vi "(alter)Mecanum Steering.vi"() -> ()   [LabVIEW 2015]
doc: "This example shows how to use the Steering VIs to define and simulate a dynamic model of a three-wheeled omnidirectional robot on a smooth surface."
uses:
  Program Files (x86)/National Instruments/LabVIEW 2015/examples/robotics/Steering/3D Omni Robot/Robot Position.ctl
  <vilib>/robotics/Steering/Wheel/Wheel Parameters.ctl
  <vilib>/robotics/Steering/Wheel/Rotation Direction.ctl
  <vilib>/Simulation/Scripting/Companion Diagram/SimConfigNode/SimParams.ctl
  <vilib>/Simulation/Scripting/Companion Diagram/SimConfigNode/_simSolvers.ctl
  <vilib>/Simulation/Implementation/Shared/SIMSCR Execution Mode.ctl
  <vilib>/Platform/TimedLoop/XDataNode/timing_clust.ctl
  <vilib>/Platform/TimedLoop/XDataNode/nitl_modes.ctl
  <vilib>/Platform/TimedLoop/XDataNode/wakeup.ctl
  <vilib>/Simulation/Param Hierarchy/Typedefs/SIMPH Param Control Actions.ctl
  <vilib>/Simulation/Implementation/Shared/NILVSim_ParamChanged.vi
  <vilib>/Simulation/Implementation/Shared/NILVSim_FinishedLate.vi
  <vilib>/Simulation/Implementation/Shared/NILVSIM_BeginStep.vi
  <vilib>/Simulation/Utility/Implementation/SIM Halt.vi
  <vilib>/Simulation/Implementation/Shared/NILVSim_Manager.vi
  <vilib>/Utility/error.llb/Clear Errors.vi
  <vilib>/Simulation/Implementation/Shared/NILVSim_FinalizeModel.vi
  <vilib>/Analysis/coordinate.llb/2D Cartesian Coordinate Rotation.vi
  <vilib>/Analysis/coordinate.llb/2D Cartesian Coordinate Rotation (Scalar).vi
  <vilib>/robotics/Steering/Omnidirectional Wheel/Create Omnidirectional Wheel.vi
  <vilib>/robotics/Steering/Steering Frame/Create User Defined Steering Frame.vi
  <vilib>/Simulation/Implementation/Shared/SIM Unbundle Sim Info.vi
  <vilib>/Simulation/Implementation/Shared/SIMSH Read Queue.vi
  <vilib>/Simulation/Implementation/Shared/NILVSim_Initialize.vi
  <vilib>/Simulation/Utility/Implementation/NILVSim Get Time and IsAcceptedStep.vi
  <vilib>/Simulation/Implementation/Shared/NILVSim_GetModelError.vi
  <vilib>/Simulation/Implementation/Shared/SIM Bundle Sim Info.vi
  <vilib>/robotics/Steering/Steering Frame/Apply Steering Frame Velocity to Motors.vi
  <vilib>/robotics/Steering/Steering Frame/Get Steering Frame Velocity from Motors.vi
  <vilib>/Simulation/Scripting/Companion Diagram/SimConfigNode/SimDog.xnode
  Program Files (x86)/National Instruments/LabVIEW 2015/examples/robotics/Steering/3D Omni Robot/Omni Robot Model.vi
  <vilib>/Platform/TimedLoop/XDataNode/XDataNode.xnode
  <vilib>/Simulation/Implementation/XNodeFramework/SimXNode/SimX.xnode
  <vilib>/robotics/Steering/Steering Frame/NI_Robotics_Steering Frame.lvclass
  <vilib>/robotics/Steering/Wheel/NI_Robotics_Wheel.lvclass
  <vilib>/robotics/Steering/Omnidirectional Wheel/NI_Robotics_Omnidirectional Wheel.lvclass
  <vilib>/Platform/TimedLoop/XDataNode/XDNodeRunTimeDep.lvlib
  <vilib>/Simulation/Implementation/Shared/NI_SIM_Implementation.lvlib
panel:
  in  "目標in 2":T1={"起始"=0.0, "終點"=200.0, "max speed(估算)"=80.0, "dt"=10.0}
  out "距離曲線(cm) 2":dbl[](array[numeric])
  out "次數 2":i32
  out "speed曲線(cm/s) 2":dbl[](array[numeric])
  out "speed曲線(cm/s)":dbl[](array[numeric])
  out "次數":i32
  out "距離曲線(cm)":dbl[](array[numeric])
  in  "目標in":T1={"起始"=0.0, "終點"=200.0, "max speed(估算)"=80.0, "dt"=10.0}
  out "Waveform Chart 2":T2(graph)
  out "xy theta":T2(graph)
  in  "Velocity":T3(ring)
  in  "reset":bool
  in  "stop":bool
  in  "Angular Velocity (rad/s)":dbl(slide) min=-7.0 max=7.0 scale=-7.0..7.0
  out "Angular Velocity Feedback":dbl(slide) scale=1.0..-1.0
  in  "Y Velocity (cm/s)":dbl(slide) min=-100.0 max=100.0 scale=-100.0..100.0
  out "Y Velocity Feedback":dbl(slide) scale=-1.0..1.0
  in  "X Velocity (cm/s)":dbl(slide) min=-100.0 max=100.0 scale=-100.0..100.0
  out "X Velocity Feedback":dbl(slide) scale=-1.0..1.0
  out "motor states":dbl[](array[numeric]) format="%#.3f"
  in  "motor setpoints":dbl[](array[numeric])=[0.0, 0.0, 0.0] format="%#.3f"
  out "complete":bool
  out "robot position":T4 {"ccw wheel angles" format="%#.3f"; "global theta" format="%#.3f"; "global y" format="%#.3f"; "global x" format="%#.3f"}
  out "3D Picture":refnum<vi>(3d-picture)
  # "This VI simulates the steering of a three-wheeled omnidirectional robot on a smooth surface.\n\n1. Run the VI, then move the sliders to control the forward, lateral, and angular velocity components of the robot.\n\n2. Press the Reset Position button to move the robot back to its starting position."
types:
  T1 = cluster{"起始":dbl, "終點":dbl, "max speed(估算)":dbl, "dt":dbl}
  T2 = cluster{"motor states[0]":dbl, "motor states[1]":dbl, "motor states[2]":dbl, "motor states[3]":dbl, "motor states[4]":dbl, "motor states[5]":dbl, "motor states[6]":dbl, "motor states[7]":dbl, "motor states[8]":dbl}
  T3 = enum16{"Relative to Steering Frame", "Relative to Global Frame"}
  T4 = typedef "Robot Position.ctl" = cluster{"global x":dbl, "global y":dbl, "global theta":dbl, "ccw wheel angles":dbl[]}
  T5 = typedef "NI_Robotics_Wheel.lvclass/Rotation Direction.ctl" = u16
  T6 = typedef "NI_Robotics_Wheel.lvclass/Wheel Parameters.ctl" = cluster{"wheel radius":dbl, "gear ratio":dbl, "forward rotation direction":T5}
  T7 = cluster{"[0]":dbl, "[1]":dbl, "[2]":dbl, "[3]":dbl, "[4]":dbl, "[5]":dbl, "[6]":dbl, "[7]":dbl, "[8]":dbl}
  T8 = typedef "SIMSCR Execution Mode.ctl" = enum16{"Simulate to Completion", "Single Time-Step Simulation (Fixed Step Only)"}
  T9 = typedef "XDNodeRunTimeDep.lvlib/timing_clust.ctl" = cluster{"Expected End [f-1]":u64, "Actual End [f-1]":u64, "Finished Late? [f-1]":bool, "Expected End [i-1]":u64, "Actual End [i-1]":u64, "Finished Late? [i-1]":bool, "Expected Start [i]":u64, "Actual Start [i]":u64, "Expected Start [f]":u64, "Actual Start [f]":u64, "Source Name":string, "Structure Name":string, "Period":i64, "Deadline":i64, "Offset":i64, "Start":i64, "Priority":i32, "Timeout":i32, "Mode":T10, "Wakeup Reason":T11, "Error":errorcluster, "Source Type":string, "Secondary Source Type":string, "Global End Time":u64, "Global Start Time":u64, "Frame Duration":u64, "Iteration Duration":u64, "Assigned CPU":i32, "I/O Scan Engine Mode":u32}
  T10 = typedef "XDNodeRunTimeDep.lvlib/nitl_modes.ctl" = enum32{"No Change", "Process missed periods, maintain original phase", "Discard missed periods, maintain original phase", "Process missed periods, ignore original phase", "Discard missed periods, ignore original phase"}
  T11 = typedef "XDNodeRunTimeDep.lvlib/wakeup.ctl" = enum32{"Normal", "Aborted", "Asynchronous wakeup", "Timing source error", "Timed loop error", "Timeout"}
  T12 = typedef "SIMPH Param Control Actions.ctl" = enum16{"get params", "set params"}
  T13 = cluster{"SIMSH Sim Time":dbl, "Mecanum Robot Body Model.vi":cluster{"theta 2":dbl, "x,y (inertial)":dbl[], "ccw wheel angles":dbl[], "ccw wheel angular velocities":dbl[]}, "Mecanum Robot Body Model.vi - SIMSH":cluster{"SIMSH Sim Time":dbl, "w":cluster{"output":dbl}, "theta":cluster{"output":dbl}, "x'":cluster{"output":dbl[]}, "x":cluster{"output":dbl[]}, "Wheel theta":cluster{"output":dbl[]}, "Negate 5":cluster{"-x":dbl[]}, "Build Array 7":cluster{"appended array":dbl[]}, "Negate 4":cluster{"-x":dbl}, "y":dbl, "Divide 6":cluster{"x/y":dbl}, "Square Root 2":cluster{"sqrt(x)":dbl}, "Build Array 6":cluster{"appended array":dbl[]}, "Build Matrix 2":cluster{"appended array":dbl[][]}, "Build Array 5":cluster{"appended array":dbl[]}, "Multiply 2":cluster{"x*y":dbl}, "Negate 3":cluster{"-x":dbl[]}, "Add Array Elements":cluster{"sum":dbl}, "Build Matrix":cluster{"appended array":dbl[][]}, "Negate 2":cluster{"-x":dbl}, "Divide 5":cluster{"x/y":dbl}, "Square Root":cluster{"sqrt(x)":dbl}, "Build Array 4":cluster{"appended array":dbl[]}, "Build Array 3":cluster{"appended array":dbl[]}, "Subtract":cluster{"x-y":dbl}, "To Double Precision Float":cluster{"double precision float":dbl}, "Build Array 2":cluster{"appended array":dbl[]}, "Boolean To (0,1)":cluster{"0, 1":i16}, "Divide 4":cluster{"x/y":dbl[]}, "A x B.vi 3":cluster{"A x Vector":dbl[]}, "Build Array":cluster{"appended array":dbl[]}, "Multiply":cluster{"x*y":dbl}, "Index Array 2":cluster{"element":dbl}, "2D Cartesian Coordinate Rotation.vi 3":cluster{"y out":dbl, "x out":dbl}, "Divide 3":cluster{"x/y":dbl[]}, "A x B.vi":cluster{"A x Vector":dbl[]}, "Divide 2":cluster{"x/y":dbl[]}, "Replace Array Subset":cluster{"output array":dbl[]}, "Negate":cluster{"-x":dbl}, "Index Array":cluster{"element":dbl}, "2D Cartesian Coordinate Rotation.vi":cluster{"y out":dbl, "x out":dbl}, "Divide":cluster{"x/y":dbl}}, "Motor Model.vi":cluster{"motor torque":dbl[]}, "Motor Model.vi - SIMSH":cluster{"SIMSH Sim Time":dbl, "Gain":cluster{"output":dbl[]}, "Summation 2":cluster{"Result":dbl[]}, "Shaft Angle":cluster{"output":dbl[]}}, "Gain":cluster{"output":dbl[]}, "Gain 2":cluster{"output":dbl[]}, "Motor Velocity PID.vi":cluster{"DC current output":dbl[]}, "Motor Velocity PID.vi - SIMSH":cluster{"SIMSH Sim Time":dbl, "Integrator":cluster{"output":dbl[]}, "Gain":cluster{"output":dbl[]}, "Summation":cluster{"Result":dbl[]}, "Derivative":cluster{"output":dbl[]}, "Saturation":cluster{"output":dbl[]}, "Build Array":cluster{"appended array":dbl[]}, "Negate 2":cluster{"-x":dbl[]}, "Absolute Value":cluster{"abs(x)":dbl[]}, "DC current max":dbl, "Multiply":cluster{"x*y":dbl[]}, "Negate":cluster{"-x":dbl[]}, "Subtract":cluster{"x-y":dbl[]}, "Divide":cluster{"x/y":dbl[]}}, "reset":bool, "Index Array":cluster{"element":dbl}, "Bundle By Name":cluster{"output cluster":cluster{"global x":dbl, "global y":dbl, "global theta":dbl, "ccw wheel angles":dbl[]}}}
  T14 = typedef "SimParams.ctl" = cluster{"Initial Time (s)":dbl, "Final Time (s)":dbl, "Step Size (s)":dbl, "ODE Solver":T15, "Minimum Step Size (s)":dbl, "Maximum Step Size (s)":dbl, "Relative Tolerance":dbl, "Absolute Tolerance":dbl, "Software Timing":bool, "Initial Step Size (s)":dbl, "Automatic Fixed Step Size?":bool, "Automatic Discrete Step Size?":bool, "Discrete Step Size (s)":dbl, "Calculate using Time Step":bool, "Solver Wired?":bool, "Prev.Frm.Expected End":u64, "Prev.Frm.Actual End":u64, "Prev.Frm.Finished Late?":bool, "Prev.Iter.Expected End":u64, "Prev.Iter.Actual End":u64, "Prev.Iter.Finished Late?":bool, "Expected Iteration Start":u64, "Actual Iteration Start":u64, "Expected Frame Start":u64, "Actual Frame Start":u64, "Source Name":string, "Name":string, "Period":i64, "Deadline":i64, "Offset":i64, "Start":i64, "Priority":i32, "Timeout":i32, "Processor":i32, "Mode":enum32{"No Change", "Process missed periods, maintain original phase", "Discard missed periods, maintain original phase", "Process missed periods, ignore original phase", "Discard missed periods, ignore original phase"}, "Wakeup reason":enum32{"Normal", "Aborted", "Asynchronous wakeup", "Timing source error", "Timed loop error", "Timeout"}, "Error":errorcluster, "Source Type":string, "Secondary Source Type":string, "Global End Time":u64, "Global Start Time":u64, "Full Solver Reset":bool, "Execution Mode":T8, "Nan/Inf Check":bool, "Custom Solver Library":string, "Solver Is Variable":bool, "custom solver name":string, "Signal Collection Decimation":u32}
  T15 = typedef "_simSolvers.ctl" = enum16{"Runge-Kutta 1 (Euler)", "Runge-Kutta 2", "Runge-Kutta 3", "Runge-Kutta 4", "Runge-Kutta 23 (variable)", "Runge-Kutta 45 (variable)", "BDF (variable)", "Adams-Moulton (variable)", "Rosenbrock (variable)", "Discrete States Only", "SDIRK 4 (variable)", "Radau 5 (variable)", "Radau 9 (variable)", "Radau 13 (variable)", "Radau [Variable Order] (variable)", "Gear's Method (variable)", "Linearizer", "State Query", "Trim Eval", "Custom Solver"}
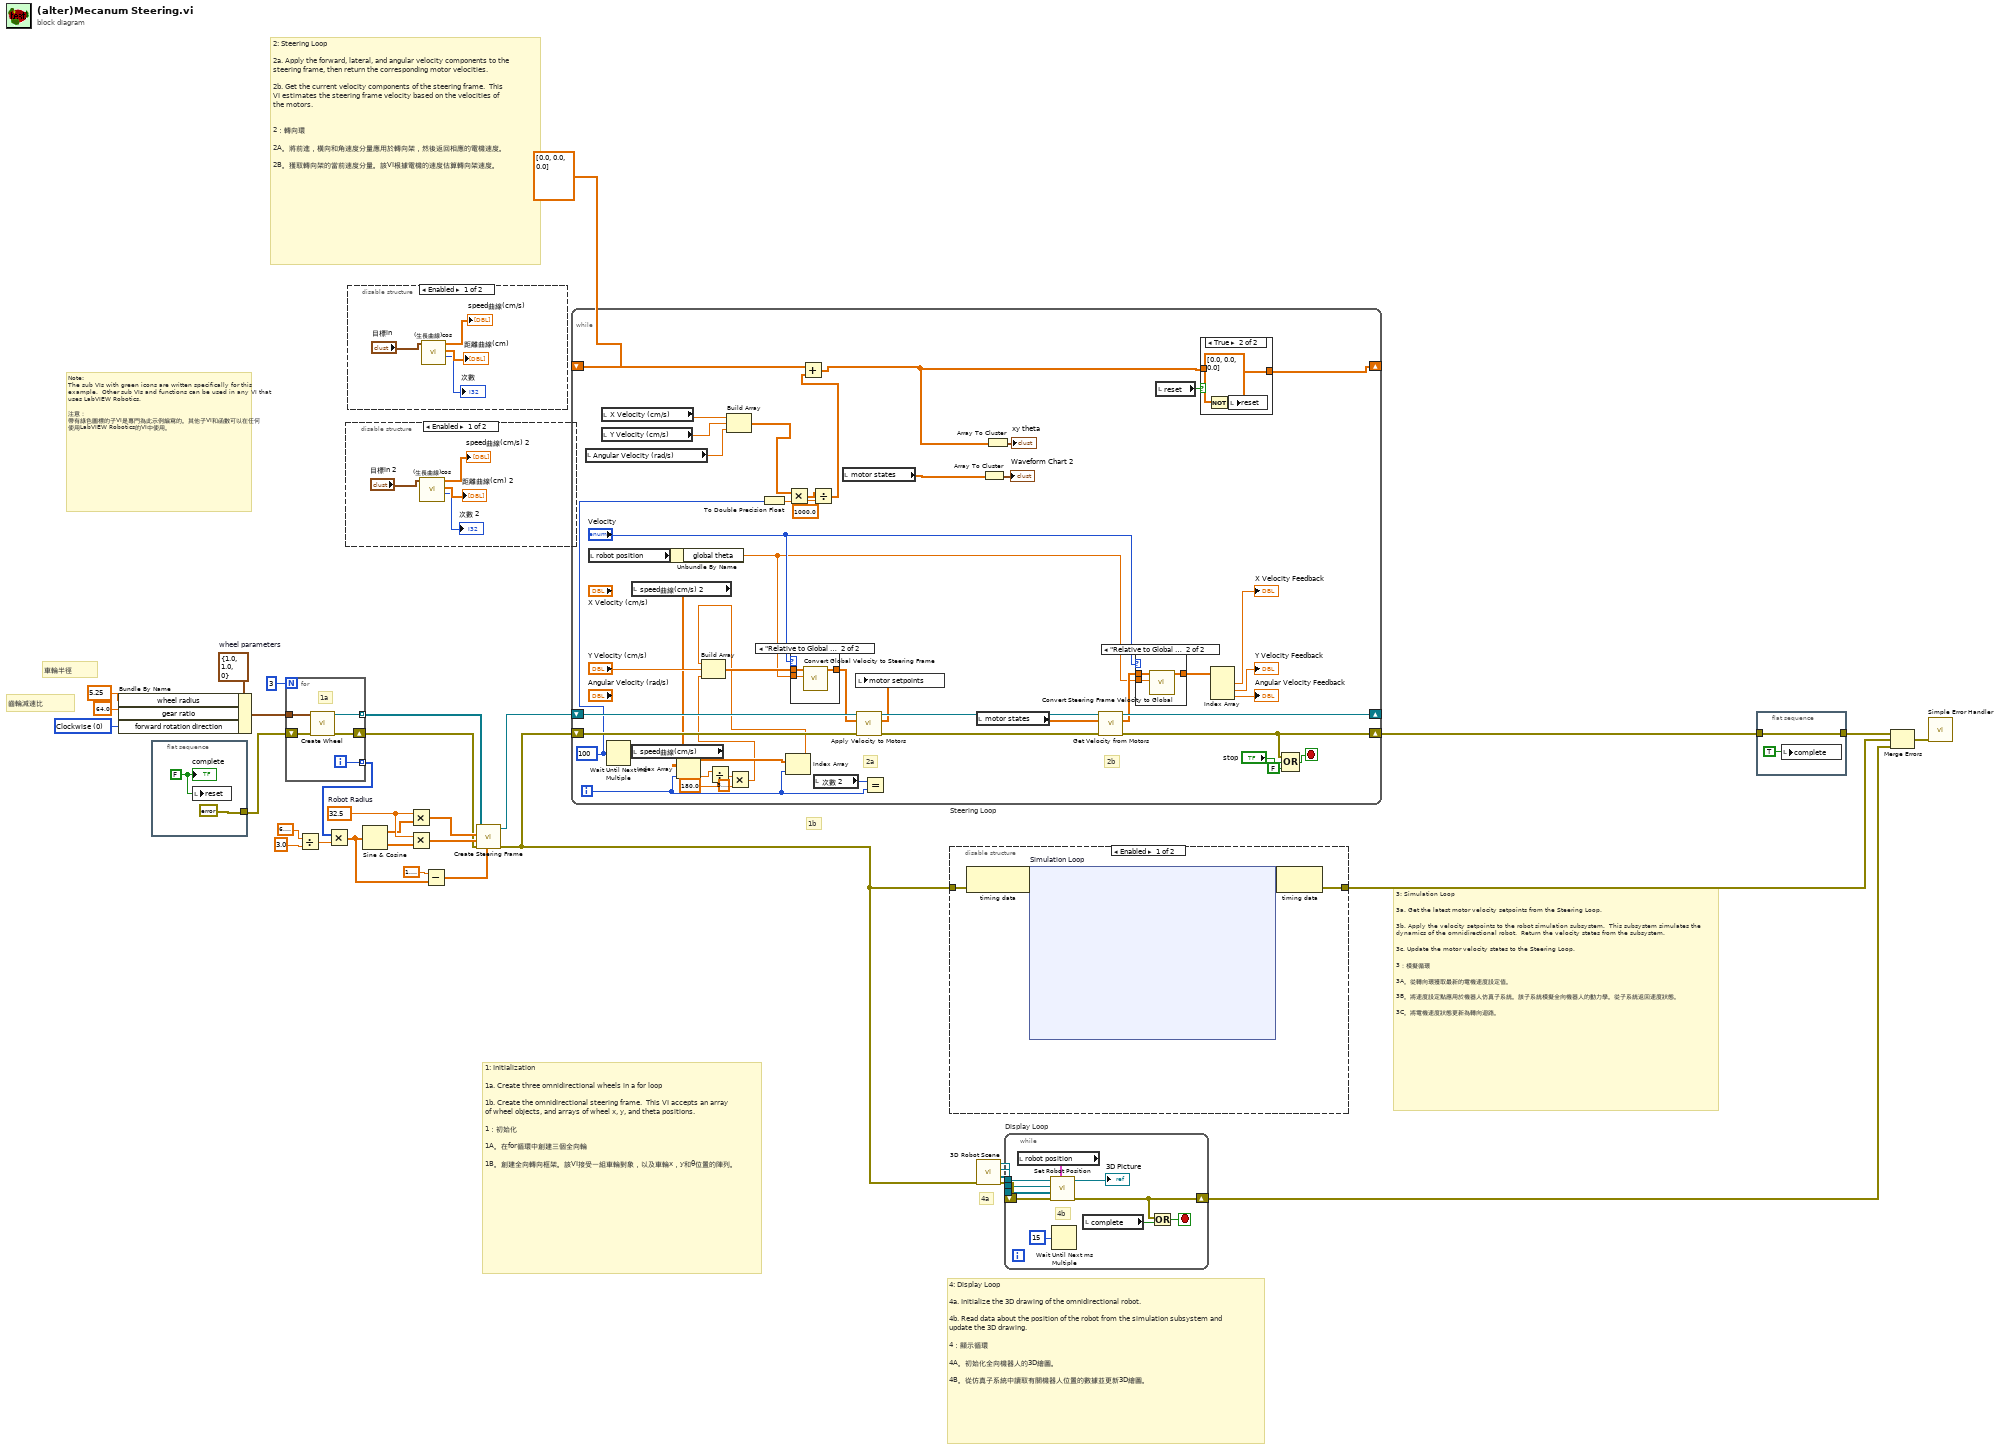
[diagram p0: block diagram]
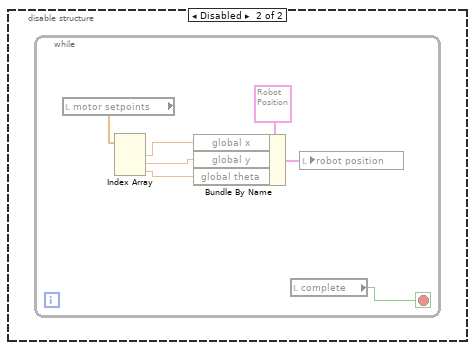
[diagram p7: hidden frame]
diagram:
  w9 = T5 0 items=["Clockwise", "Counterclockwise"] ("forward rotation direction")
  w14 = 32.5  # Robot Radius
  w32 = T6 {"wheel radius"=1.0, "gear ratio"=1.0, "forward rotation direction"=0}  # wheel parameters
  # "齒輪減速比"
  # "車輪半徑"
  # "3: Simulation Loop\n\n3a. Get the latest motor velocity setpoints from the Steering Loop.\n\n3b. Apply the velocity setpoints to the robot simulation subsystem.  This subsystem simulates the dynamics of the omnidirectional robot.  Return the velocity states from the subsystem.\n\n3c. Update the motor velocity states to the Steering Loop.\n\n3：模擬循環\n\n3A。從轉向環獲取最新的電機速度設定值。\n\n3B。將速度設定點應用於機器人仿真子系統。該子系統模擬全向機器人的動力學。從子系統返回速度狀態。\n\n3C。將電機速度狀態更新為轉向迴路。"
  # "Note:\nThe sub VIs with green icons are written specifically for this example.  Other sub VIs and functions can be used in any VI that uses LabVIEW Robotics.\n\n注意：\n帶有綠色圖標的子VI是專門為此示例編寫的。其他子VI和函數可以在任何使用LabVIEW Robotics的VI中使用。"
  # "4a"
  # "4: Display Loop\n\n4a. Initialize the 3D drawing of the omnidirectional robot.\n\n4b. Read data about the position of the robot from the simulation subsystem and update the 3D drawing.\n\n4：顯示循環\n\n4A。初始化全向機器人的3D繪圖。\n\n4B。從仿真子系統中讀取有關機器人位置的數據並更新3D繪圖。"
  # "2: Steering Loop\n\n2a. Apply the forward, lateral, and angular velocity components to the steering frame, then return the corresponding motor velocities.\n\n2b. Get the current velocity components of the steering frame.  This VI estimates the steering frame velocity based on the velocities of the motors.\n\n\n2：轉向環\n\n2A。將前進，橫向和角速度分量應用於轉向架，然後返回相應的電機速度。\n\n2B。獲取轉向架的當前速度分量。該VI根據電機的速度估算轉向架速度。"
  # "1b"
  # "1: Initialization\n\n1a. Create three omnidirectional wheels in a for loop\n\n1b. Create the omnidirectional steering frame.  This VI accepts an array of wheel objects, and arrays of wheel x, y, and theta positions.\n\n1：初始化\n\n1A。在for循環中創建三個全向輪\n\n1B。創建全向轉向框架。該VI接受一組車輪對象，以及車輪x，y和θ位置的陣列。"
  n1 = Bundle By Name(cluster=w32, "wheel radius"=5.25, "gear ratio"=64.0, "forward rotation direction"=w9) -> (w29:T6)
  n2 = flat-sequence {
    tunnel: [errorcluster {"status"=FALSE, "code"=0, "source"=""} ("error out")] -> w24
    frame #0 {
      w34 = FALSE ("complete")
      n3 = local write "reset"(w34) -> ()
      "complete" <- w34
    }
  }
  n4 = for {
    N: 3 -> [_]
    shift-right: [w39] -> w6
    shift-left: w24 -> [w40]
    tunnel: [w38] -> w19 mode=indexing
    tunnel: w29 -> [w37]
    tunnel: [w36] -> w15 mode=indexing
    i -> [w36]
    # "1a"
    n5 = call-poly <vilib>:"Create Wheel.vi"("error in (no error)"=w40, "wheel parameters"=w37) -> ("error out"=w39:errorcluster, "omni wheel out"=w38:refnum<class "NI_Robotics_Omnidirectional Wheel.lvclass">)  [unwired: 8 in]
  }
  n6 = Divide(x=6.283185307179586, y=3.0) -> (x/y=w16:dbl)
  n7 = Multiply(x=w15, y=w16) -> (x*y=w5:dbl[])
  n8 = disable-structure shown="Enabled" {
    frame Enabled {
      n9 = call "(生長曲線)cos.vi"("目標in"="目標in 2") -> ("次數"=→"次數 2":i32, "距離曲線(cm)"=→"距離曲線(cm) 2":dbl[], "speed曲線(cm/s)"=→"speed曲線(cm/s) 2":dbl[])  [unwired: 8 in]
    }
    frame Disabled {
    }
  }
  n10 = disable-structure shown="Enabled" {
    frame Enabled {
      n11 = call "(生長曲線)cos.vi"("目標in"="目標in") -> ("次數"=→"次數":i32, "距離曲線(cm)"=→"距離曲線(cm)":dbl[], "speed曲線(cm/s)"=→"speed曲線(cm/s)":dbl[])  [unwired: 8 in]
    }
    frame Disabled {
    }
  }
  n12 = Sine & Cosine(0:w5) -> (1:w4:dbl[], 2:w3:dbl[])
  n13 = Multiply(x=w14, y=w4) -> (x*y=w13:dbl[])
  n14 = Multiply(x=w14, y=w3) -> (x*y=w12:dbl[])
  n15 = Subtract(x=1.5707963267948966, y=w5) -> (x-y=w10:dbl[])
  n16 = call-poly <vilib>:"Create Steering Frame.vi"("wheel frame angles (rad)"=w10, "error in (no error)"=w6, "wheel y positions"=w12, "wheel x positions"=w13, "wheels"=w19) -> ("error out"=w1:errorcluster, "steering frame out"=w33:refnum<class "NI_Robotics_Steering Frame.lvclass">)  [unwired: 5 in]
  n17 = while "Steering Loop" {
    shift-right: [w88] -> _
    shift-left: w33 -> [w91]
    shift-right: [w61] -> w25
    shift-left: w1 -> [w90]
    shift-right: [w70] -> _
    shift-left: dbl[] [0.0, 0.0, 0.0] -> [w79]
    i -> [w57]
    stop <- w62 stop-if-true
    w69 = u32 100 ("millisecond multiple")
    # "2b"
    # "2a"
    n18 = local read "Angular Velocity (rad/s)"() -> (w78:dbl)
    n19 = local read "robot position"() -> (w82:T4)
    n20 = local read "X Velocity (cm/s)"() -> (w76:dbl)
    n21 = local read "Y Velocity (cm/s)"() -> (w77:dbl)
    n22 = Wait Until Next ms Multiple(millisecond multiple=w69) -> ()  [unwired: 1 out]
    n23 = local read "speed曲線(cm/s) 2"() -> (w58:dbl[])
    n24 = local read "speed曲線(cm/s)"() -> (w63:dbl[])
    n25 = Unbundle By Name(w82) -> ("global theta"=w81:dbl)
    n26 = Index Array(array=w63, index=w57) -> (element=w54:dbl)
    n27 = Divide(x=w54, y=180.0) -> (x/y=w52:dbl)
    n28 = Build Array(w76, w77, w78) -> (w68:dbl[])
    n29 = Multiply(x=w52, y=3.141592653589793) -> (x*y=w49:dbl)
    n30 = To Double Precision Float(number=w69) -> (double precision float=w66:dbl)
    n31 = Index Array(array=w58, index=w57) -> (element=w56:dbl)
    n32 = Build Array(w56, "Y Velocity (cm/s)", w49) -> (w85:dbl[])
    n33 = Multiply(x=w68, y=w66) -> (x*y=w67:dbl[])
    n34 = case shown="\"Relative to Global Frame\"" "Velocity" {
      tunnel: w85 -> [w105 w108]
      tunnel: [w105 w107] -> w80
      tunnel: w81 -> [_ w106]
      frame "Relative to Steering Frame", Default {
      }
      frame "Relative to Global Frame" {
        n35 = call <vilib>:"Convert Global Velocity to Steering Frame.vi"("steering frame angle (rad)"=w106, "global velocity"=w108) -> ("steering frame velocity"=w107:dbl[])  [unwired: 9 in]
      }
    }
    n36 = Divide(x=w67, y=1000.0) -> (x/y=w64:dbl[])
    n37 = Add(x=w79, y=w64) -> (x+y=w71:dbl[])
    n38 = local read "次數 2"() -> (w59:i32)
    n39 = local read "motor states"() -> (w74:dbl[])
    n40 = call-poly <vilib>:"Apply Velocity to Motors.vi"("error in (no error)"=w90, "steering frame velocity"=w80, "steering frame in"=w91) -> ("error out"=w89:errorcluster, "ccw motor velocity setpoints"=w50:dbl[], "steering frame out"=w92:refnum<class "NI_Robotics_Steering Frame.lvclass">)  [unwired: 4 in, 2 out]
    n41 = local write "motor setpoints"(w50) -> ()
    n42 = Equal?(x=w59, y=w57) -> ()  [unwired: 1 out]
    n43 = local read "motor states"() -> (w87:dbl[])
    n44 = Array To Cluster(array=w74) -> (cluster=→"Waveform Chart 2":T2)
    n45 = Array To Cluster(array=w71) -> (cluster=→"xy theta":T7)
    n46 = call-poly <vilib>:"Get Velocity from Motors.vi"("error in (no error)"=w89, "ccw motor velocity states"=w87, "steering frame in"=w92) -> ("error out"=w61:errorcluster, "estimated steering frame velocity"=w84:dbl[], "steering frame out"=w88:refnum<class "NI_Robotics_Steering Frame.lvclass">)  [unwired: 6 in]
    n47 = case shown="\"Relative to Global Frame\"" "Velocity" {
      tunnel: w84 -> [w101 w104]
      tunnel: [w101 w103] -> w83
      tunnel: w81 -> [_ w102]
      frame "Relative to Steering Frame", Default {
      }
      frame "Relative to Global Frame" {
        n48 = call <vilib>:"Convert Steering Frame Velocity to Global.vi"("steering frame angle (rad)"=w102, "steering frame velocity"=w104) -> ("global velocity"=w103:dbl[])  [unwired: 9 in]
      }
    }
    n49 = local read "reset"() -> (w72:bool)
    n50 = case shown="True" w72 {
      selector: w72 -> [_ w98]
      tunnel: w71 -> [w97 _]
      tunnel: [w97 dbl[] [0.0, 0.0, 0.0]] -> w70
      frame False {
      }
      frame True {
        n51 = Not(x=w98) -> (.not. x?=w99:bool)
        n52 = local write "reset"(w99) -> ()
      }
    }
    n53 = Index Array(array=w83) -> (element #1=→"X Velocity Feedback":dbl, element #2=→"Y Velocity Feedback":dbl, element #3=→"Angular Velocity Feedback":dbl)  [unwired: 3 in]
    n54 = Compound Arithmetic op=OR(w61, "stop", FALSE ("value")) -> (w62:bool)
  }
  n55 = disable-structure shown="Enabled" {
    disable-tunnel: [w110 _] -> w7
    disable-tunnel: w1 -> [w109 _]
    frame Enabled {
      n56 = node-c288(w109) -> (w112:variant)
      n57 = node-c254 "Simulation Loop"(w112) -> (w111:variant)
      n58 = node-c288(w111) -> (w110:errorcluster)
    }
    frame Disabled {
      n59 = while {
        stop <- w399 stop-if-true
        n60 = local read "motor setpoints"() -> (w404:dbl[])
        n61 = Index Array(array=w404) -> (element #1=w403:dbl, element #2=w402:dbl, element #3=w401:dbl)  [unwired: 3 in]
        n62 = Bundle By Name(cluster=T4 {"global x"=0.0, "global y"=0.0, "global theta"=5.186146767450741, "ccw wheel angles"=[-12.965366918626874, -12.965366918626874, -12.965366918626874]} ("robot position 2"), "global x"=w403, "global y"=w402, "global theta"=w401) -> (w400:T4)
        n63 = local read "complete"() -> (w399:bool)
        n64 = local write "robot position"(w400) -> ()
      }
    }
  }
  n65 = call "3D Robot Scene.vi"("error in (no error)"=w1) -> ("error out"=w21:errorcluster, "axles"=w26:refnum<vi>[], "robot"=w27:refnum<vi>, "scene"=w28:refnum<vi>)  [unwired: 7 in]
  n66 = while "Display Loop" {
    tunnel: w28 -> [w409]
    tunnel: w27 -> [w410]
    tunnel: w26 -> [w411]
    shift-right: [w406] -> w20
    shift-left: w21 -> [w412]
    stop <- w407 stop-if-true
    # "4b"
    n67 = local read "robot position"() -> (w413:T4)
    n68 = call "Set Robot Position.vi"("robot position"=w413, "error in (no error)"=w412, "axles"=w411, "robot"=w410, "scene"=w409) -> ("error out"=w406:errorcluster, "scene out"=→"3D Picture":refnum<vi>)  [unwired: 5 in]
    n69 = Wait Until Next ms Multiple(millisecond multiple=u32 15) -> ()  [unwired: 1 out]
    n70 = local read "complete"() -> (w408:bool)
    n71 = Or(x=w406, y=w408) -> (x .or. y?=w407:bool)
  }
  n72 = flat-sequence {
    tunnel: w25 -> [w416]
    tunnel: [w416] -> w23
    frame #0 {
      n73 = local write "complete"(TRUE ("complete")) -> ()
    }
  }
  n74 = Merge Errors(w23, w7, w20) -> (w22:errorcluster)
  n75 = call <vilib>:"Simple Error Handler.vi"("error in (no error)"=w22) -> ()  [unwired: 4 in, 5 out]
